vi "eeprom test.vi"() -> ()   [LabVIEW 2009]
uses:
  <vilib>/Instr/_visa.llb/VISA Configure Serial Port (Instr).vi
panel:
  out "write buffer length":string
  out "Loop Count":i32
  out "bytes read":u32
  in  "measure wait time":bool=TRUE
  out "send string":string
  in  "store write buffer in eeprom":bool
  in  "write buffer":string
  in  "string to send":string="t\u0002\u0000E "
  in  "Retrys":i32=1
  out "Average serial wait":dbl
  out "wait time":u32
  out "bytes written":u32
  out "read buffer":string
  in  "VISA resource name":refnum<visa-resource-name>
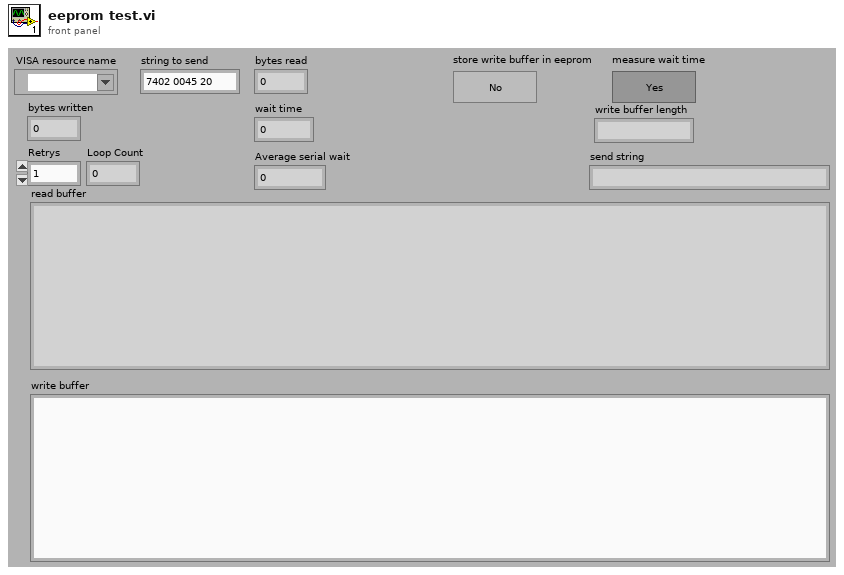
[diagram p1: front panel]
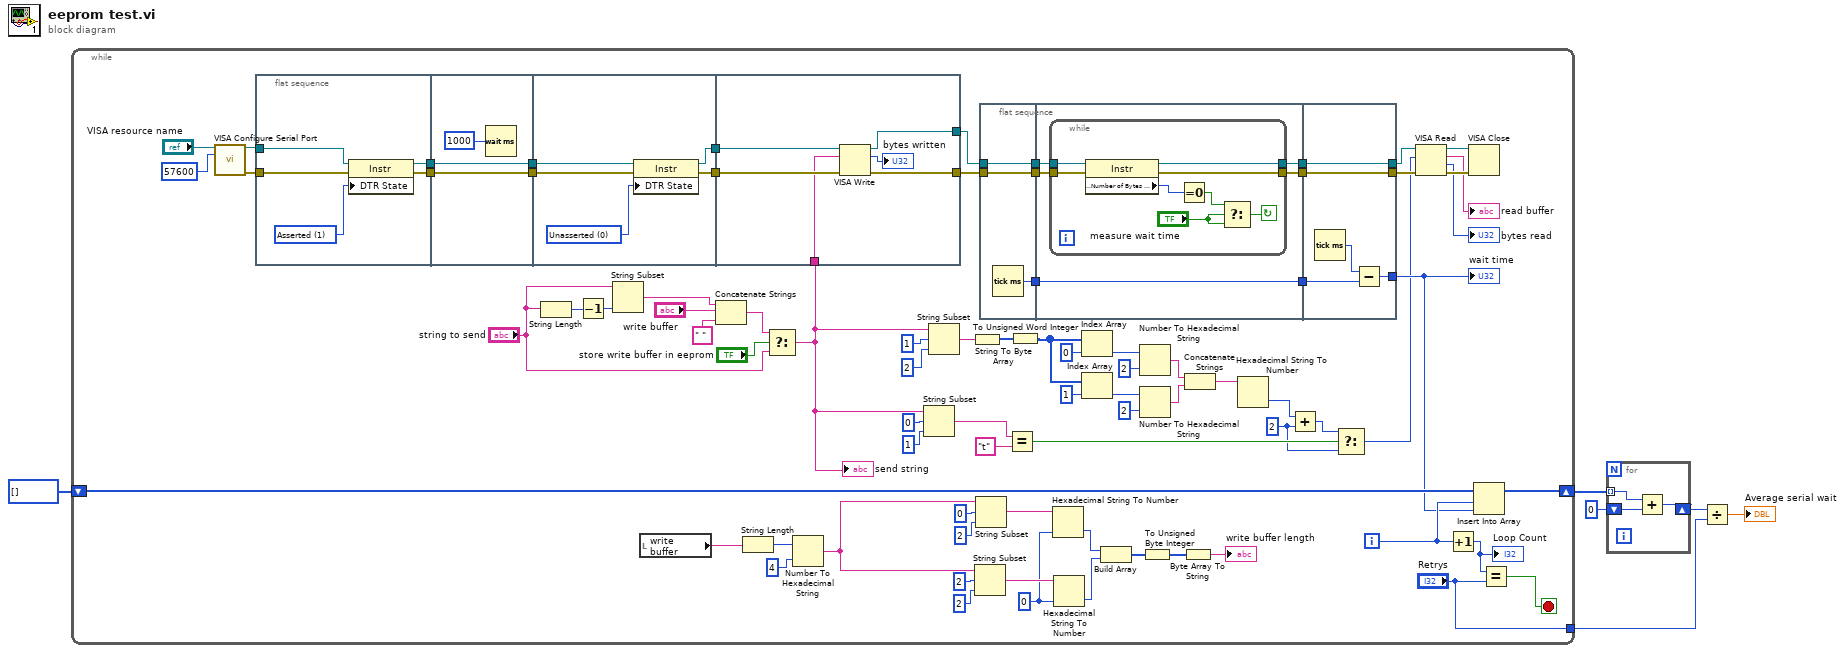
[diagram p0: block diagram]
diagram:
  n1 = while {
    shift-right: [w85] -> w5
    shift-left: u32[] [] -> [w84]
    tunnel: ["Retrys"] -> w1
    i -> [w80]
    stop <- w83 stop-if-true
    w13 = u16 0 ("default (0 U32)")
    w24 = u32 2 ("y")
    n2 = call-poly "VISA Configure Serial Port"("VISA resource name"="VISA resource name", "baud rate (9600)"=u32 57600 ("baud rate")) -> ("VISA resource name out"=w57:refnum<visa-resource-name>, "error out"=w56:errorcluster)  [unwired: 12 in]
    n3 = flat-sequence {
      tunnel: w57 -> [w111]
      tunnel: w56 -> [w110]
      tunnel: [w109] -> w71
      tunnel: [w108] -> w70
      tunnel: w71 -> [w114]
      tunnel: w70 -> [w113]
      tunnel: [w114] -> w69
      tunnel: [w113] -> w68
      tunnel: w69 -> [w118]
      tunnel: w68 -> [w115]
      tunnel: [w117] -> w67
      tunnel: [w116] -> w66
      tunnel: w67 -> [w124]
      tunnel: w66 -> [w123]
      tunnel: w29 -> [w120]
      tunnel: [w122] -> w61
      tunnel: [w121] -> w60
      frame #0 {
        w107 = i16 1 items=["Unknown"=-1, "Unasserted"=0, "Asserted"=1] ("Serial Settings:Modem Line Settings:Line RTS State")
        n4 = property class="Instr"(reference=w111, error in=w110, "DTR State"=w107) -> (reference out=w109:refnum<visa-resource-name>, error out=w108:errorcluster)
      }
      frame #1 {
        n5 = Wait (ms)(milliseconds to wait=u32 1000) -> ()  [unwired: 1 out]
      }
      frame #2 {
        w119 = i16 0 items=["Unknown"=-1, "Unasserted"=0, "Asserted"=1] ("Serial Settings:Modem Line Settings:Line RTS State")
        n6 = property class="Instr"(reference=w118, error in=w115, "DTR State"=w119) -> (reference out=w117:refnum<visa-resource-name>, error out=w116:errorcluster)
      }
      frame #3 {
        n7 = VISA Write(VISA resource name=w124, write buffer=w120, error in (no error)=w123) -> (VISA resource name out=w122:refnum<visa-resource-name>, return count=→"bytes written":u32, error out=w121:errorcluster)
      }
    }
    n8 = String Length(string="string to send") -> (length=w77:i32)
    n9 = Decrement(x=w77) -> (x-1=w78:i32)
    n10 = String Subset(string="string to send", length (rest)=w78) -> (substring=w74:string)  [unwired: 1 in]
    n11 = local read "write buffer"() -> (w22:string)
    n12 = Concatenate Strings(w74, "write buffer", " ") -> (w75:string)
    n13 = String Length(string=w22) -> (length=w21:i32)
    n14 = Select(t=w75, s="store write buffer in eeprom", f="string to send") -> (s? t:f=w29:string)
    "send string" <- w29
    n15 = Number To Hexadecimal String(1:i16 4 ("width (-)"), 2:w21) -> (0:w16:string)
    n16 = String Subset(string=w29, offset (0)=0, length (rest)=1 ("length (rest)")) -> (substring=w27:string)
    n17 = String Subset(string=w29, offset (0)=1 ("length (rest)"), length (rest)=2 ("length (rest)")) -> (substring=w44:string)
    n18 = String To Byte Array(string=w44) -> (unsigned byte array=w41:u8[])
    n19 = String Subset(string=w16, offset (0)=2, length (rest)=2 ("length (rest)")) -> (substring=w14:string)
    n20 = String Subset(string=w16, offset (0)=0, length (rest)=2 ("length (rest)")) -> (substring=w15:string)
    n21 = flat-sequence {
      tunnel: w60 -> [w87]
      tunnel: w61 -> [w88]
      tunnel: [w88] -> w53
      tunnel: [w87] -> w52
      tunnel: [w86] -> w50
      tunnel: [w93] -> w55
      tunnel: [w92] -> w54
      tunnel: w53 -> [w91]
      tunnel: w52 -> [w90]
      tunnel: [w89] -> w51
      tunnel: w50 -> [w89]
      tunnel: [w105] -> w47
      tunnel: [w106] -> w48
      tunnel: w55 -> [w106]
      tunnel: w54 -> [w105]
      tunnel: w51 -> [w103]
      tunnel: [w102] -> w49
      frame #0 {
        n22 = Tick Count (ms)() -> (millisecond timer value=w86:u32)
      }
      frame #1 {
        n23 = while {
          tunnel: [w101] -> w93
          tunnel: [w100] -> w92
          tunnel: w91 -> [w99]
          tunnel: w90 -> [w98]
          stop <- w94 continue-if-true
          n24 = property class="Instr"(reference=w99, error in=w98) -> (reference out=w101:refnum<visa-resource-name>, error out=w100:errorcluster, "Serial Settings:Number of Bytes at Serial Port"=w97:u32)
          n25 = Equal To 0?(x=w97) -> (x = 0?=w95:bool)
          n26 = Select(t=w95, s="measure wait time", f="measure wait time") -> (s? t:f=w94:bool)
        }
      }
      frame #2 {
        n27 = Tick Count (ms)() -> (millisecond timer value=w104:u32)
        n28 = Subtract(x=w104, y=w103) -> (x-y=w102:u32)
      }
    }
    n29 = Equal?(x=w27, y="t") -> (x = y?=w25:bool)
    n30 = To Unsigned Word Integer(number=w41) -> (unsigned 16bit integer=w40:u16[])
    n31 = Hexadecimal String To Number(string=w15, default (0uL)=w13) -> (number=w12:u16)  [unwired: 1 in, 1 out]
    n32 = Hexadecimal String To Number(string=w14, default (0uL)=w13) -> (number=w11:u16)  [unwired: 1 in, 1 out]
    n33 = Index Array(array=w40, index=0) -> (element=w39:u16)
    n34 = Index Array(array=w40, index=1) -> (element=w38:u16)
    n35 = Build Array(w12, w11) -> (w10:u16[])
    n36 = Number To Hexadecimal String(1:i16 2 ("width (-)"), 2:w39) -> (0:w34:string)
    n37 = Number To Hexadecimal String(1:i16 2 ("width (-)"), 2:w38) -> (0:w33:string)
    n38 = To Unsigned Byte Integer(number=w10) -> (unsigned 8bit integer=w9:u8[])
    n39 = Byte Array To String(unsigned byte array=w9) -> (string=→"write buffer length":string)
    n40 = Concatenate Strings(w34, w33) -> (w35:string)
    n41 = Hexadecimal String To Number(string=w35) -> (number=w32:u32)  [unwired: 2 in, 1 out]
    n42 = Add(x=w32, y=w24) -> (x+y=w30:u32)
    n43 = Select(t=w30, s=w25, f=w24) -> (s? t:f=w31:u32)
    n44 = VISA Read(VISA resource name=w48, byte count=w31, error in (no error)=w47) -> (VISA resource name out=w64:refnum<visa-resource-name>, read buffer=→"read buffer":string, return count=→"bytes read":u32, error out=w63:errorcluster)
    n45 = Increment(x=w80) -> (x+1=w81:i32)
    "Loop Count" <- w81
    n46 = VISA Close(VISA resource name=w64, error in (no error)=w63) -> ()  [unwired: 1 out]
    n47 = Insert Into Array(array=w84, index=w80, new element=w49) -> (w85:u32[])
    n48 = Equal?(x=w81, y="Retrys") -> (x = y?=w83:bool)
    "wait time" <- w49
  }
  n49 = for {
    tunnel: w5 -> [w128] mode=indexing
    shift-right: [w126] -> w3
    shift-left: u32 0 -> [w127]
    n50 = Add(x=w128, y=w127) -> (x+y=w126:u32)
  }
  n51 = Divide(x=w3, y=w1) -> (x/y=→"Average serial wait":dbl)
